vi "init.vi"(9 "Hash Function":refnum<vi>, 10 "Bucket Size":u32, 11 "NumBuckets":i32) -> (0 "error out":errorcluster, 3 "HashMap out":refnum<class "HashMap.lvclass">)   [LabVIEW 2017, in "HashMap.lvclass"]
uses:
  <userlib>/836-Library/Data_Structures/HashMap/HashMap.lvclass
  <userlib>/836-Library/Data_Structures/HashMap/HashMap.lvclass/HashMap.ctl
  <vilib>/Utility/error.llb/Error Cluster From Error Code.vi
  <vilib>/ErrorRing/Error Ring.xnode
  <userlib>/836-Library/Data_Structures/Bucket/Bucket.lvclass
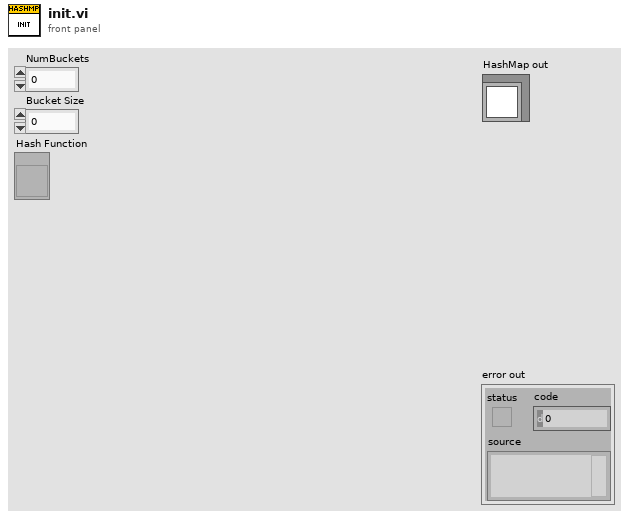
[diagram p1: front panel]
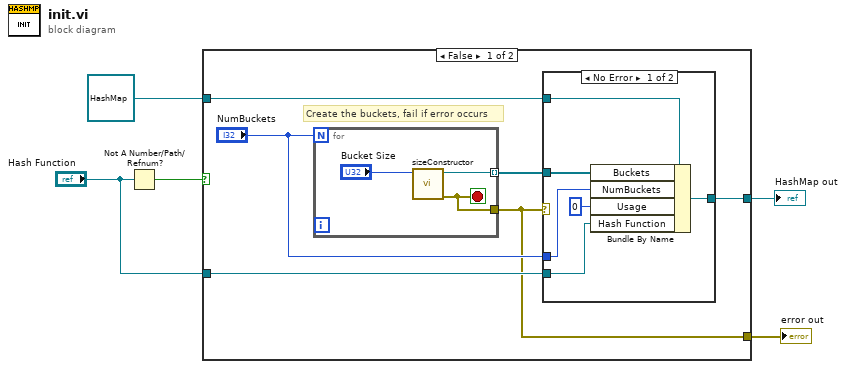
[diagram p0: block diagram]
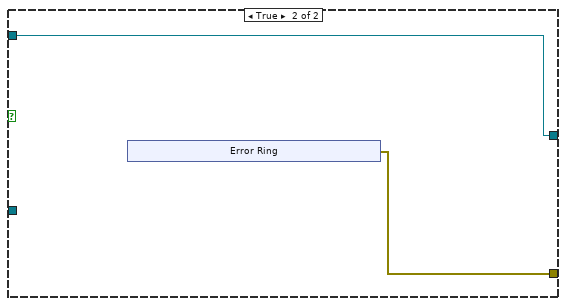
[diagram p3: hidden frame]
diagram:
  n1 = Not A Number/Path/Refnum?(number/path/refnum="Hash Function") -> (NaN/Path/Refnum?=w5:bool)
  n2 = case shown="False" w5 {
    tunnel: "Hash Function" -> [w7 _]
    tunnel: refnum<class "HashMap.lvclass"> refnum ("HashMap out") -> [w10 w23]
    tunnel: [w9 w23] -> w2
    tunnel: [w6 w22] -> w1
    frame False {
      # "Create the buckets, fail if error occurs"
      n3 = for {
        N: "NumBuckets" -> [_]
        tunnel: [w20] -> w11 mode=indexing
        tunnel: [w19] -> w6
        stop <- w19 stop-if-true
        n4 = call <userlib>:"sizeConstructor.vi"("Size"="Bucket Size") -> ("error out"=w19:errorcluster, "Bucket out"=w20:refnum<class "Bucket.lvclass">)  [unwired: 9 in]
      }
      n5 = case shown="No Error" w6 {
        tunnel: w11 -> [w17 _]
        tunnel: w10 -> [w16 w18]
        tunnel: [w15 w18] -> w9
        tunnel: "NumBuckets" -> [w14 _]
        tunnel: w7 -> [w12 _]
        frame No Error {
          n6 = Bundle By Name(cluster=w16, "Buckets"=w17, "NumBuckets"=w14, "Usage"=0, "Hash Function"=w12) -> (w15:refnum<class "HashMap.lvclass">)
        }
        frame Error {
        }
      }
    }
    frame True {
      n7 = xnode "Error Ring"() -> ("error out"=w22:errorcluster)
    }
  }
  "error out" <- w1
  "HashMap out" <- w2
